vi "Part 1.vi"(11 "Input":string) -> (3 "Output":i64)   [LabVIEW 2021]
uses:
  <userlib>/_OpenG.lib/string/string.llb/Convert EOLs (String)__ogtk.vi
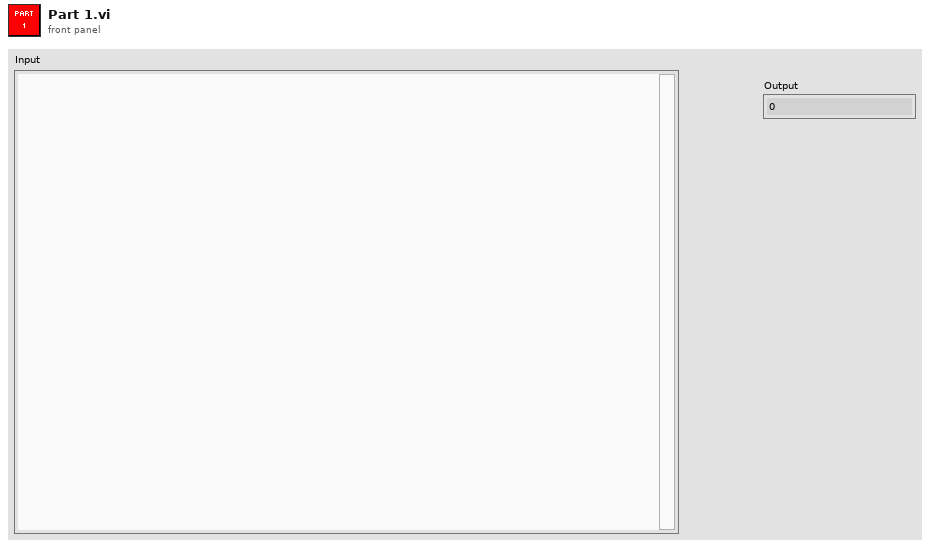
[diagram p1: front panel]
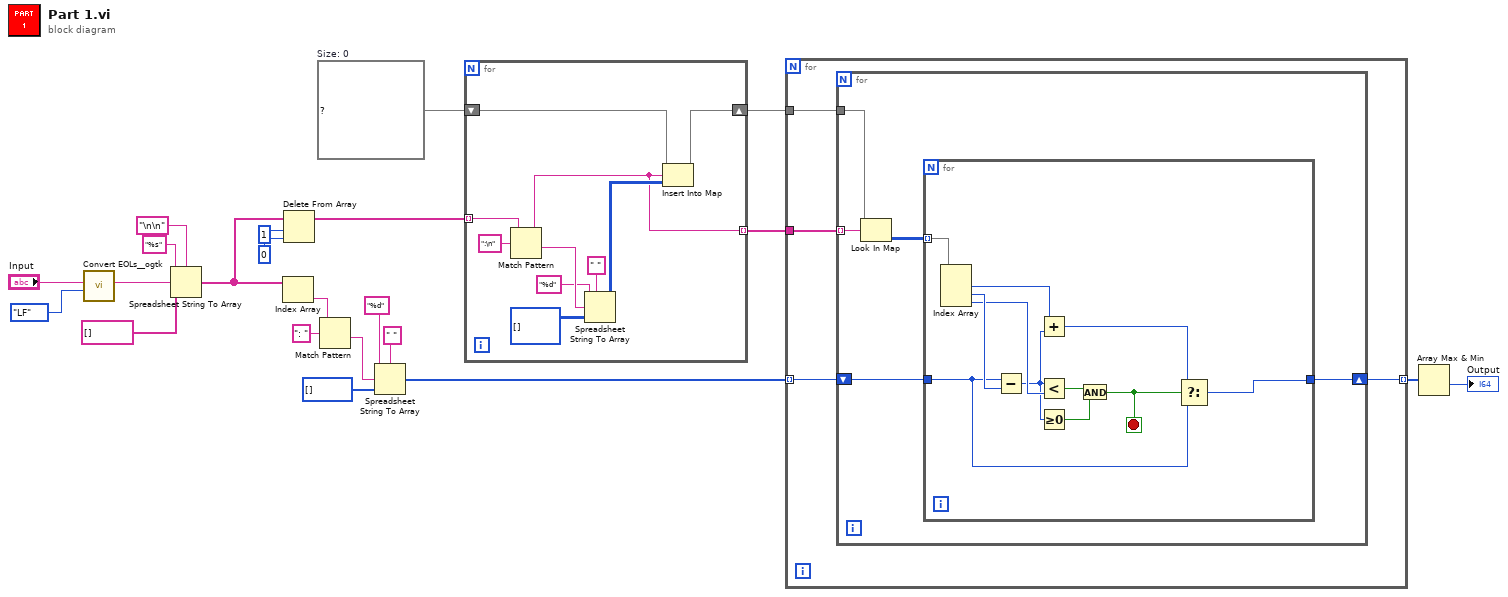
[diagram p0: block diagram]
diagram:
  w7 = map{string, i64[][]} {}  # Size: 0
  n1 = call-poly <userlib>:"Convert EOLs__ogtk.vi"("Convert to:"=enum16{"CR", "LF", "CRLF"}."LF", "String in"="Input") -> ("String out"=w18:string)  [unwired: 9 in]
  n2 = Spreadsheet String To Array(delimiter (Tab)="\n\n", format string="%s", spreadsheet string=w18, array type (2D Dbl)=string[] []) -> (array=w13:string[])
  n3 = Index Array(array=w13) -> (element=w12:string)  [unwired: 1 in]
  n4 = Delete From Array(array=w13, length=1, index=0) -> (array with subset deleted=w15:string[])  [unwired: 1 out]
  n5 = Match Pattern(string=w12, regular expression=": " ("search string/char (-)")) -> (after substring=w9:string)  [unwired: 1 in, 3 out]
  n6 = Spreadsheet String To Array(delimiter (Tab)=" ", format string="%d", spreadsheet string=w9, array type (2D Dbl)=i64[] []) -> (array=w6:i64[])
  n7 = for {
    tunnel: w15 -> [w31] mode=indexing
    shift-right: [w24] -> w4
    shift-left: w7 -> [w26]
    tunnel: [w23] -> w5 mode=indexing
    n8 = Match Pattern(string=w31, regular expression=":\n" ("search string/char (-)")) -> (before substring=w23:string, after substring=w29:string)  [unwired: 1 in, 2 out]
    n9 = Spreadsheet String To Array(delimiter (Tab)=" ", format string="%d", spreadsheet string=w29, array type (2D Dbl)=i64[][] []) -> (array=w25:i64[][])
    n10 = Insert Into Map(map in=w26, key=w23, value=w25) -> (map out=w24:map{string, i64[][]})  [unwired: 2 out]
  }
  n11 = for {
    tunnel: w6 -> [w36] mode=indexing
    tunnel: w5 -> [w35]
    tunnel: w4 -> [w34]
    tunnel: [w33] -> w1 mode=indexing
    n12 = for {
      tunnel: w35 -> [w41] mode=indexing
      tunnel: w34 -> [w40]
      shift-right: [w37] -> w33
      shift-left: w36 -> [w38]
      n13 = Look In Map(map=w40, key=w41) -> (value=w39:i64[][])  [unwired: 1 in, 1 out]
      n14 = for {
        tunnel: w39 -> [w52] mode=indexing
        tunnel: w38 -> [w44]
        tunnel: [w42] -> w37
        stop <- w45 stop-if-true
        n15 = Index Array(array=w52) -> (element #1=w46:i64, element #2=w51:i64, element #3=w50:i64)  [unwired: 3 in]
        n16 = Subtract(x=w44, y=w51) -> (x-y=w47:i64)
        n17 = Add(x=w46, y=w47) -> (x+y=w43:i64)
        n18 = Less?(x=w47, y=w50) -> (x < y?=w49:bool)
        n19 = Greater Or Equal To 0?(x=w47) -> (x >= 0?=w48:bool)
        n20 = And(x=w49, y=w48) -> (x .and. y?=w45:bool)
        n21 = Select(t=w43, s=w45, f=w44) -> (s? t:f=w42:i64)
      }
    }
  }
  n22 = Array Max & Min(array=w1) -> (min value=→"Output":i64)  [unwired: 3 out]
